vi "Remove Shared Variable.vi"(8 "error in (no error)":errorcluster, 11 "Node Ptr":u64 format="%.0x") -> (0 "error out":errorcluster)   [LabVIEW 2017, in "Shared Variables CD 2.0 Configuration.lvlib"]
uses:
  Shared Variables CD 2.0 Configuration.lvlib
  Support/ChannelVS/ChannelVS.lvclass
  Support/ChannelVS/ChannelVS.lvclass/ChannelVS.ctl
panel:
  in  "Tag":string
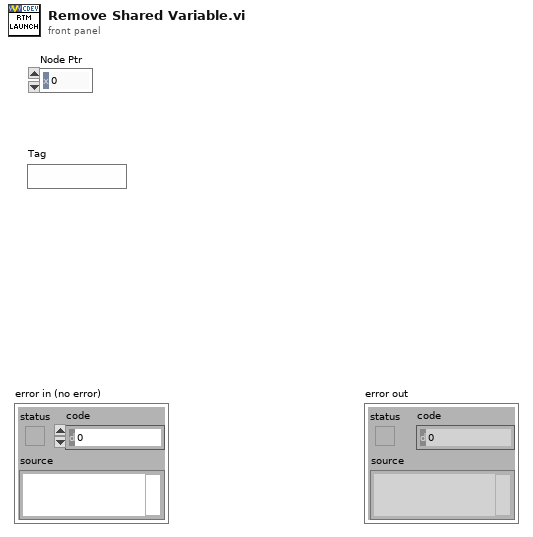
[diagram p1: front panel]
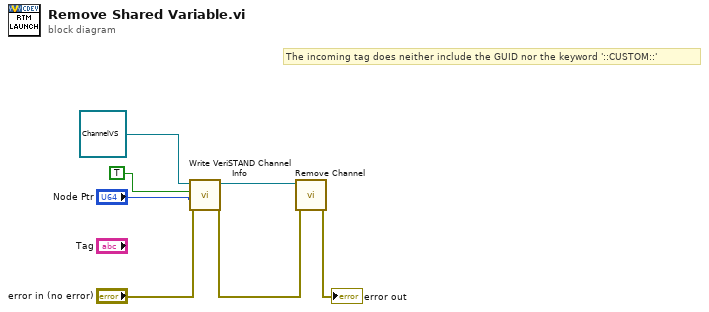
[diagram p0: block diagram]
diagram:
  # "The incoming tag does neither include the GUID nor the keyword '::CUSTOM::'"
  n1 = call "Write VeriSTAND Channel Info.vi"("error in (no error)"="error in (no error)", "VeriSTAND Reference"="Node Ptr", "Exist in VeriSTAND"=TRUE ("Exists in VS?"), "ChannelVS in"=refnum<class "ChannelVS.lvclass"> refnum ("Shared Variables CD 2.0 Configuration.lvlib:ChannelVS.lvclass")) -> ("error out"=w5:errorcluster, "ChannelVS out"=w1:refnum<class "ChannelVS.lvclass">)  [unwired: 6 in]
  n2 = call "Remove Channel.vi"("error in (no error)"=w5, "ChannelVS in"=w1) -> ("error out"=→"error out":errorcluster)  [unwired: 8 in, 1 out]
